vi "Quit.vi"(8 "No Error":errorcluster) -> (0 "error out":errorcluster)   [LabVIEW 2026, in "SDL3.lvlib" / "TTF.lvlib"]
doc: "<B>Summary</B>\nDeinitialize SDL_ttf.\n\n<B>Remarks</B>\nYou must call this when done with the library, to free internal resources. It is safe to call this when the library isn't initialized, as it will just return immediately.\n\nOnce you have as many quit calls as you have had successful calls to <B>TTF_Init</B>, the library will actually deinitialize.\n\nPlease note that this does not automatically close any fonts that are still open at the time of deinitialization, and it is possibly not safe to close them afterwards, as parts of the library will no longer be initialized to deal with it. A well-written program should call <B>TTF_CloseFont()</B> on any open fonts before calling this function!"
uses:
  TTF.lvlib
  Lib/SDL3_ttf.dll
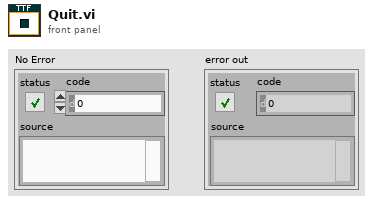
[diagram p1: front panel]
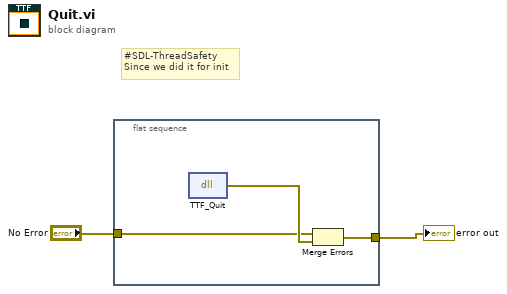
[diagram p0: block diagram]
diagram:
  # "#SDL-ThreadSafety\nSince we did it for init"
  n1 = flat-sequence {
    tunnel: [w4] -> w2
    tunnel: "No Error" -> [w3]
    frame #0 {
      n2 = dll-call lib="C:/Users/saukko/Dev/LV-SDL3/Sources/SDL3/Lib/SDL3_ttf.*" fn="TTF_Quit"() -> (error out=w5:errorcluster)  [unwired: 4 in, 1 out]
      n3 = Merge Errors(w3, w5) -> (w4:errorcluster)
    }
  }
  "error out" <- w2
